vi "Input_Scale_v00.vi"(11 "Control":T7={"PII In 1"={"Lock"=FALSE, "Hold"=FALSE, "P Gain"=0, "P BS"=-5, "I Gain"=0, "I BS"=-10, "I2 G"=0, "I2 BS"=-26, "Scan Amp"=0, "Scan Off"=0, "Scan FS"=0, "SFS BS"=0, "I Max value"=10000, "I2 Max value"=10000, "Scope.Offset"=0, "Trigger Direction"=enum."either", "Scan-PII thresh"=0}, "PII In 2"={"Lock"=FALSE, "Hold"=FALSE, "P Gain"=0, "P BS"=-10, "I Gain"=0, "I BS"=-10, "I2 G"=0, "I2 BS"=-26, "Scan Amp"=0, "Scan Off"=0, "Scan FS"=0, "SFS BS"=0, "I Max value"=10000, "I2 Max value"=10000, "Scope.Offset"=0, "Trigger Direction"=enum."either", "Scan-PII thresh"=0}, "PII In 3"={"Lock"=FALSE, "Hold"=FALSE, "P Gain"=0, "P BS"=-10, "I Gain"=0, "I BS"=-10, "I2 G"=0, "I2 BS"=-26, "Scan Amp"=0, "Scan Off"=0, "Scan FS"=0, "SFS BS"=0, "I Max value"=10000, "I2 Max value"=10000, "Scope.Offset"=0, "Trigger Direction"=enum."either", "Scan-PII thresh"=0}, "PII In 4"={"Lock"=FALSE, "Hold"=FALSE, "P Gain"=0, "P BS"=-10, "I Gain"=0, "I BS"=-10, "I2 G"=0, "I2 BS"=-26, "Scan Amp"=0, "Scan Off"=0, "Scan FS"=0, "SFS BS"=0, "I Max value"=10000, "I2 Max value"=10000, "Scope.Offset"=0, "Trigger Direction"=enum."either", "Scan-PII thresh"=0}, "Safety First"={"lim reset"=FALSE, "no limit"=FALSE, "pos slew rate * dt"=10, "neg slew rate * dt"=-10, "Hold All"=FALSE, "Count(Ticks)"=0}, "Error scale"={"Pre-Offset"={"Pre-Offset 1"=2, "Pre-Offset 2"=0, "Pre-Offset 3"=0, "Pre-Offset 4"=0, "Pre-Offset 5"=2, "Pre-Offset 6"=0, "Pre-Offset 7"=0, "Pre-Offset 8"=0}, "Post-Offset "={"Offset 1"=0, "Offset 2"=300, "Offset 3"=0, "Offset 4"=0, "Offset 5"=0, "Offset 6"=0, "Offset 7"=0, "Offset 8"=0}, "Gains"={"Gain 1"=0, "Gain 2"=300, "Gain 3"=0, "Gain 4"=0, "Gain 5"=0, "Gain 6"=0, "Gain 7"=0, "Gain 8"=0}, "Polarity DC"={"False 1"=FALSE, "False 2"=FALSE, "False 3"=FALSE, "False 4"=FALSE, "DC x -1"=FALSE, "DC x -1 2"=FALSE, "DC x -1 3"=FALSE, "DC x -1 4"=FALSE}}, "Lock Thresh"={"OPO A"=2, "OPO B"=0, "MCC"=40, "Doubler"=0}, "Re-Scan Thresh"={"OPO A"=0, "OPO B"=0, "MCC"=0, "Doubler"=0}}) -> (3 "Signals":T1={"Cavity Errors"={"OPO A"=0, "OPO B"=0, "MCC"=0, "Doubler"=0}, "Cavity Monitors"={"OPO A Monitor"=0, "OPO B Monitor"=0, "MCC Monitor"=0, "Doubler Monitor"=0}, "Lock Thresh"={"OPO A"=0, "OPO B"=0, "MCC"=0, "Doubler"=0}, "Re-Scan Thresh"={"OPO A"=0, "OPO B"=0, "MCC"=0, "Doubler"=0}, "PII In 1"={"Lock"=FALSE, "Hold"=FALSE, "P Gain"=0, "P BS"=-5, "I Gain"=0, "I BS"=-10, "I2 G"=0, "I2 BS"=-26, "Scan Amp"=0, "Scan Off"=0, "Scan FS"=0, "SFS BS"=0, "I Max value"=10000, "I2 Max value"=10000, "Scope.Offset"=0, "Trigger Direction"=enum."either", "Scan-PII thresh"=0}, "PII In 2"={"Lock"=FALSE, "Hold"=FALSE, "P Gain"=0, "P BS"=-10, "I Gain"=0, "I BS"=-10, "I2 G"=0, "I2 BS"=-26, "Scan Amp"=0, "Scan Off"=0, "Scan FS"=0, "SFS BS"=0, "I Max value"=10000, "I2 Max value"=10000, "Scope.Offset"=0, "Trigger Direction"=enum."either", "Scan-PII thresh"=0}, "PII In 3"={"Lock"=FALSE, "Hold"=FALSE, "P Gain"=0, "P BS"=-10, "I Gain"=0, "I BS"=-10, "I2 G"=0, "I2 BS"=-26, "Scan Amp"=0, "Scan Off"=0, "Scan FS"=0, "SFS BS"=0, "I Max value"=10000, "I2 Max value"=10000, "Scope.Offset"=0, "Trigger Direction"=enum."either", "Scan-PII thresh"=0}, "PII In 4"={"Lock"=FALSE, "Hold"=FALSE, "P Gain"=0, "P BS"=-10, "I Gain"=0, "I BS"=-10, "I2 G"=0, "I2 BS"=-26, "Scan Amp"=0, "Scan Off"=0, "Scan FS"=0, "SFS BS"=0, "I Max value"=10000, "I2 Max value"=10000, "Scope.Offset"=0, "Trigger Direction"=enum."either", "Scan-PII thresh"=0}, "Safety First"={"lim reset"=FALSE, "no limit"=FALSE, "pos slew rate * dt"=10, "neg slew rate * dt"=-10, "Hold All"=FALSE, "Count(Ticks)"=0}})   [LabVIEW 2010]
doc: "Reads in and scales the 8 FPGA inputs. Bundles the signals as 4 cavity error signals and 4 cavity DC monitors."
uses:
  Strict Type Defs/FPGA Inputs.ctl
  Strict Type Defs/Cavity Monitors.ctl
  Strict Type Defs/Control.ctl
  Strict Type Defs/PII individual.ctl
  Strict Type Defs/Safety First.ctl
  Strict Type Defs/Error Scale.ctl
  Strict Type Defs/Lock Thresh.ctl
  Strict Type Defs/Signals.ctl
  Strict Type Defs/Cavity Errors.ctl
  <vilib>/eio/EIONode/EIONode.xnode
  <vilib>/rvi/eio/nirviEIOImplementation/nirviEIOImplementation.xnode
  <vilib>/rvi/eio/common/nirviEmuClasses.ctl
  <vilib>/rvi/eio/common/nirviEmuTemplateMethod_noerrors.vi
panel:
  in  "Signals":T1={"Cavity Errors"={"OPO A"=0, "OPO B"=0, "MCC"=0, "Doubler"=0}, "Cavity Monitors"={"OPO A Monitor"=0, "OPO B Monitor"=0, "MCC Monitor"=0, "Doubler Monitor"=0}, "Lock Thresh"={"OPO A"=0, "OPO B"=0, "MCC"=0, "Doubler"=0}, "Re-Scan Thresh"={"OPO A"=0, "OPO B"=0, "MCC"=0, "Doubler"=0}, "PII In 1"={"Lock"=FALSE, "Hold"=FALSE, "P Gain"=0, "P BS"=-5, "I Gain"=0, "I BS"=-10, "I2 G"=0, "I2 BS"=-26, "Scan Amp"=0, "Scan Off"=0, "Scan FS"=0, "SFS BS"=0, "I Max value"=10000, "I2 Max value"=10000, "Scope.Offset"=0, "Trigger Direction"=enum."either", "Scan-PII thresh"=0}, "PII In 2"={"Lock"=FALSE, "Hold"=FALSE, "P Gain"=0, "P BS"=-10, "I Gain"=0, "I BS"=-10, "I2 G"=0, "I2 BS"=-26, "Scan Amp"=0, "Scan Off"=0, "Scan FS"=0, "SFS BS"=0, "I Max value"=10000, "I2 Max value"=10000, "Scope.Offset"=0, "Trigger Direction"=enum."either", "Scan-PII thresh"=0}, "PII In 3"={"Lock"=FALSE, "Hold"=FALSE, "P Gain"=0, "P BS"=-10, "I Gain"=0, "I BS"=-10, "I2 G"=0, "I2 BS"=-26, "Scan Amp"=0, "Scan Off"=0, "Scan FS"=0, "SFS BS"=0, "I Max value"=10000, "I2 Max value"=10000, "Scope.Offset"=0, "Trigger Direction"=enum."either", "Scan-PII thresh"=0}, "PII In 4"={"Lock"=FALSE, "Hold"=FALSE, "P Gain"=0, "P BS"=-10, "I Gain"=0, "I BS"=-10, "I2 G"=0, "I2 BS"=-26, "Scan Amp"=0, "Scan Off"=0, "Scan FS"=0, "SFS BS"=0, "I Max value"=10000, "I2 Max value"=10000, "Scope.Offset"=0, "Trigger Direction"=enum."either", "Scan-PII thresh"=0}, "Safety First"={"lim reset"=FALSE, "no limit"=FALSE, "pos slew rate * dt"=10, "neg slew rate * dt"=-10, "Hold All"=FALSE, "Count(Ticks)"=0}}
  in  "Cavity Monitors":T3
  in  "Cavity Errors":T9
  in  "FPGA Inputs":T10
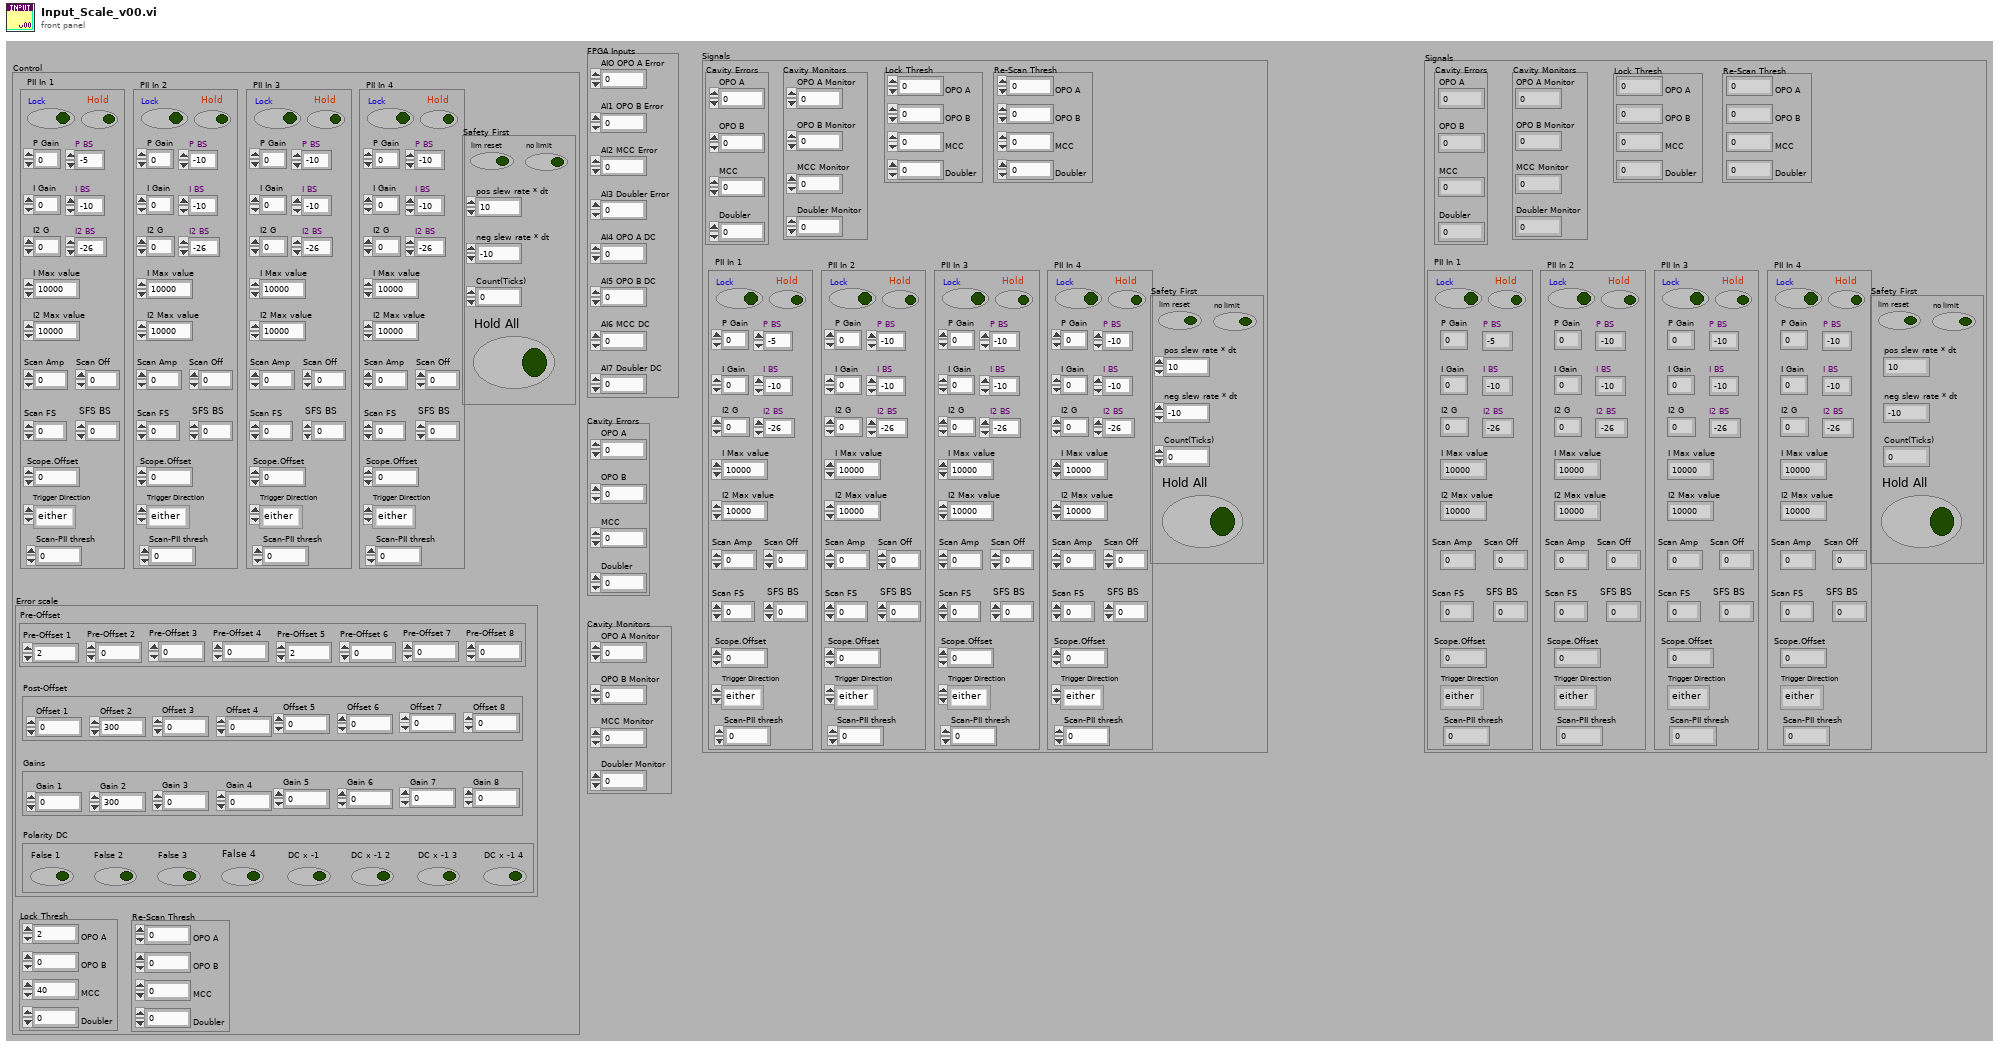
[diagram p1: front panel]
types:
  T1 = typedef "Signals.ctl" = cluster{"Cavity Errors":T2, "Cavity Monitors":T3, "Lock Thresh":T4, "Re-Scan Thresh":T4, "PII In 1":T5, "PII In 2":T5, "PII In 3":T5, "PII In 4":T5, "Safety First":T6}
  T2 = typedef "Cavity Errors.ctl" = cluster{"OPO A":i16, "OPO B":i16, "MCC":i16, "Doubler":i16}
  T3 = typedef "Cavity Monitors.ctl" = cluster{"OPO A Monitor":i16, "OPO B Monitor":i16, "MCC Monitor":i16, "Doubler Monitor":i16}
  T4 = typedef "Lock Thresh.ctl" = cluster{"OPO A":i16, "OPO B":i16, "MCC":i16, "Doubler":i16}
  T5 = typedef "PII individual.ctl" = cluster{"Lock":bool, "Hold":bool, "P Gain":i32, "P BS":i16, "I Gain":i32, "I BS":i16, "I2 G":i32, "I2 BS":i16, "Scan Amp":i16, "Scan Off":i16, "Scan FS":u16, "SFS BS":i16, "I Max value":i32, "I2 Max value":i32, "Scope.Offset":i16, "Trigger Direction":enum8{"either", "minus-plus", "plus-minus"}, "Scan-PII thresh":i16}
  T6 = typedef "Safety First.ctl" = cluster{"lim reset":bool, "no limit":bool, "pos slew rate * dt":i16, "neg slew rate * dt":i16, "Hold All":bool, "Count(Ticks)":u32}
  T7 = typedef "Control.ctl" = cluster{"PII In 1":T5, "PII In 2":T5, "PII In 3":T5, "PII In 4":T5, "Safety First":T6, "Error scale":T8, "Lock Thresh":T4, "Re-Scan Thresh":T4}
  T8 = typedef "Error Scale.ctl" = cluster{"Pre-Offset":cluster{"Pre-Offset 1":i16, "Pre-Offset 2":i16, "Pre-Offset 3":i16, "Pre-Offset 4":i16, "Pre-Offset 5":i16, "Pre-Offset 6":i16, "Pre-Offset 7":i16, "Pre-Offset 8":i16}, "Post-Offset ":cluster{"Offset 1":i16, "Offset 2":i16, "Offset 3":i16, "Offset 4":i16, "Offset 5":i16, "Offset 6":i16, "Offset 7":i16, "Offset 8":i16}, "Gains":cluster{"Gain 1":i16, "Gain 2":i16, "Gain 3":i16, "Gain 4":i16, "Gain 5":i16, "Gain 6":i16, "Gain 7":i16, "Gain 8":i16}, "Polarity DC":cluster{"False 1":bool, "False 2":bool, "False 3":bool, "False 4":bool, "DC x -1":bool, "DC x -1 2":bool, "DC x -1 3":bool, "DC x -1 4":bool}}
  T9 = cluster{"OPO A":i16, "OPO B":i16, "MCC":i16, "Doubler":i16}
  T10 = typedef "FPGA Inputs.ctl" = cluster{"AIO OPO A Error":i16, "AI1 OPO B Error":i16, "AI2 MCC Error":i16, "AI3 Doubler Error":i16, "AI4 OPO A DC":i16, "AI5 OPO B DC":i16, "AI6 MCC DC":i16, "AI7 Doubler DC":i16}
  T11 = cluster{"False 1":i16, "False 2":i16, "False 3":i16, "False 4":i16, "DC x -1":i16, "DC x -1 2":i16, "DC x -1 3":i16, "DC x -1 4":i16}
  T12 = cluster{"Offset 1":i16, "Offset 2":i16, "Offset 3":i16, "Offset 4":i16, "Offset 5":i16, "Offset 6":i16, "Offset 7":i16, "Offset 8":i16}
  T13 = cluster{"Gain 1":i16, "Gain 2":i16, "Gain 3":i16, "Gain 4":i16, "Gain 5":i16, "Gain 6":i16, "Gain 7":i16, "Gain 8":i16}
  T14 = cluster{"Pre-Offset 1":i16, "Pre-Offset 2":i16, "Pre-Offset 3":i16, "Pre-Offset 4":i16, "Pre-Offset 5":i16, "Pre-Offset 6":i16, "Pre-Offset 7":i16, "Pre-Offset 8":i16}
  T15 = cluster{"False 1":bool, "False 2":bool, "False 3":bool, "False 4":bool, "DC x -1":bool, "DC x -1 2":bool, "DC x -1 3":bool, "DC x -1 4":bool}
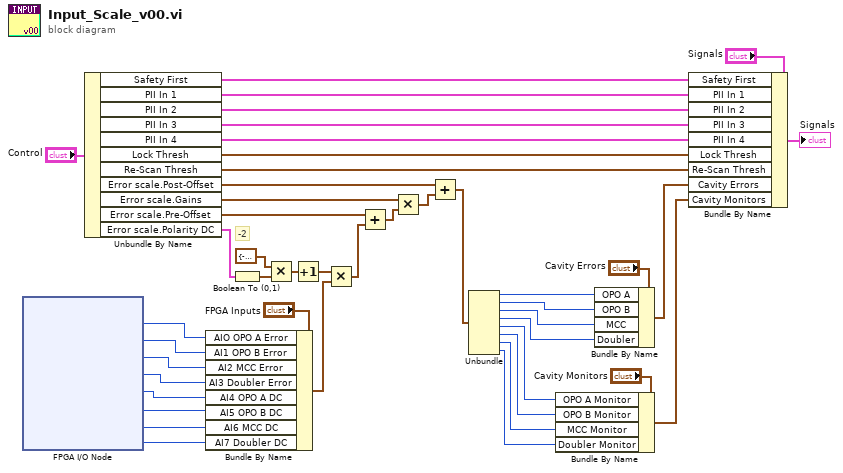
[diagram p0: block diagram]
diagram:
  # "-2"
  n1 = xnode "FPGA I/O Node"() -> ("Connector0/AI0"=w8:i16, "Connector0/AI1"=w1:i16, "Connector0/AI2"=w2:i16, "Connector0/AI3"=w3:i16, "Connector0/AI4"=w4:i16, "Connector0/AI5"=w5:i16, "Connector0/AI6"=w6:i16, "Connector0/AI7"=w7:i16)  [unwired: 8 in, 8 out]
  n2 = Unbundle By Name("Control") -> ("Safety First"=w15:T6, "PII In 1"=w14:T5, "PII In 2"=w13:T5, "PII In 3"=w12:T5, "PII In 4"=w11:T5, "Lock Thresh"=w17:T4, "Re-Scan Thresh"=w16:T4, "Error scale.Post-Offset"=w44:T12, "Error scale.Gains"=w41:T13, "Error scale.Pre-Offset"=w42:T14, "Error scale.Polarity DC"=w39:T15)
  n3 = Bundle By Name(cluster="FPGA Inputs", "AIO OPO A Error"=w8, "AI1 OPO B Error"=w1, "AI2 MCC Error"=w2, "AI3 Doubler Error"=w3, "AI4 OPO A DC"=w4, "AI5 OPO B DC"=w5, "AI6 MCC DC"=w6, "AI7 Doubler DC"=w7) -> (w22:T10)
  n4 = Boolean To (0,1)(Boolean=w39) -> (0, 1=w26:T11)
  n5 = Multiply(x=T11 {"False 1"=-2, "False 2"=-2, "False 3"=-2, "False 4"=-2, "DC x -1"=-2, "DC x -1 2"=-2, "DC x -1 3"=-2, "DC x -1 4"=-2}, y=w26) -> (x*y=w24:T11)
  n6 = Increment(x=w24) -> (x+1=w23:T11)
  n7 = Multiply(x=w23, y=w22) -> (x*y=w38:T10)
  n8 = Add(x=w42, y=w38) -> (x+y=w43:T10)
  n9 = Multiply(x=w41, y=w43) -> (x*y=w20:T10)
  n10 = Add(x=w44, y=w20) -> (x+y=w37:T10)
  n11 = Unbundle(w37) -> ("AIO OPO A Error"=w34:i16, "AI1 OPO B Error"=w33:i16, "AI2 MCC Error"=w32:i16, "AI3 Doubler Error"=w31:i16, "AI4 OPO A DC"=w30:i16, "AI5 OPO B DC"=w29:i16, "AI6 MCC DC"=w28:i16, "AI7 Doubler DC"=w27:i16)
  n12 = Bundle By Name(cluster="Cavity Monitors", "OPO A Monitor"=w30, "OPO B Monitor"=w29, "MCC Monitor"=w28, "Doubler Monitor"=w27) -> (w10:T3)
  n13 = Bundle By Name(cluster="Cavity Errors", "OPO A"=w34, "OPO B"=w33, "MCC"=w32, "Doubler"=w31) -> (w9:T9)
  n14 = Bundle By Name(cluster="Signals", "Safety First"=w15, "PII In 1"=w14, "PII In 2"=w13, "PII In 3"=w12, "PII In 4"=w11, "Lock Thresh"=w17, "Re-Scan Thresh"=w16, "Cavity Errors"=w9, "Cavity Monitors"=w10) -> (→"Signals":T1)
